vi "Sequence.CreateStepLoop.vi"(7 "Iteration":string, 8 "error in (no error)":errorcluster, 10 "Duration":dbl, 11 "Elements":T1[](array[typedef])) -> (0 "error out":errorcluster, 3 "Tasks":refnum<k24>[](array[refnum]))   [LabVIEW 2013, in "Simple Sequence Tools - Editor.lvlib"]
uses:
  Simple Sequence Tools - Editor.lvlib
  NationalInstruments.VeriStand.RealTimeSequenceDefinitionApi
  Types/Compiled.StepElementProperties.ctl
  Shared/Types/Channel.Properties.ctl
  Shared/Types/Step.Types.ctl
  Shared/SubVIs/Main.Constants.vi
  Shared/Simple Sequence Tools - Shared.lvlib
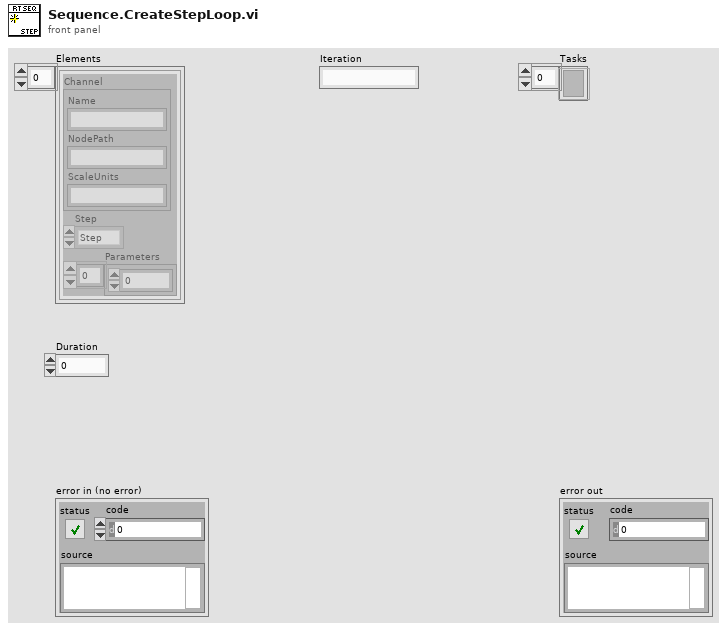
[diagram p1: front panel]
types:
  T1 = typedef "Simple Sequence Tools - Editor.lvlib/Compiled.StepElementProperties.ctl" = cluster{"Channel":T2, "Step":T3, "Parameters":dbl[]}
  T2 = typedef "Simple Sequence Tools - Shared.lvlib/Channel.Properties.ctl" = cluster{"Name":string, "NodePath":string, "ScaleUnits":string}
  T3 = typedef "Simple Sequence Tools - Shared.lvlib/Step.Types.ctl" = enum8{"Step", "iStep", "Ramp", "Unchanged", "Unknown", "Sine", "LogSine", "LinearSine", "ForcedRamp"}
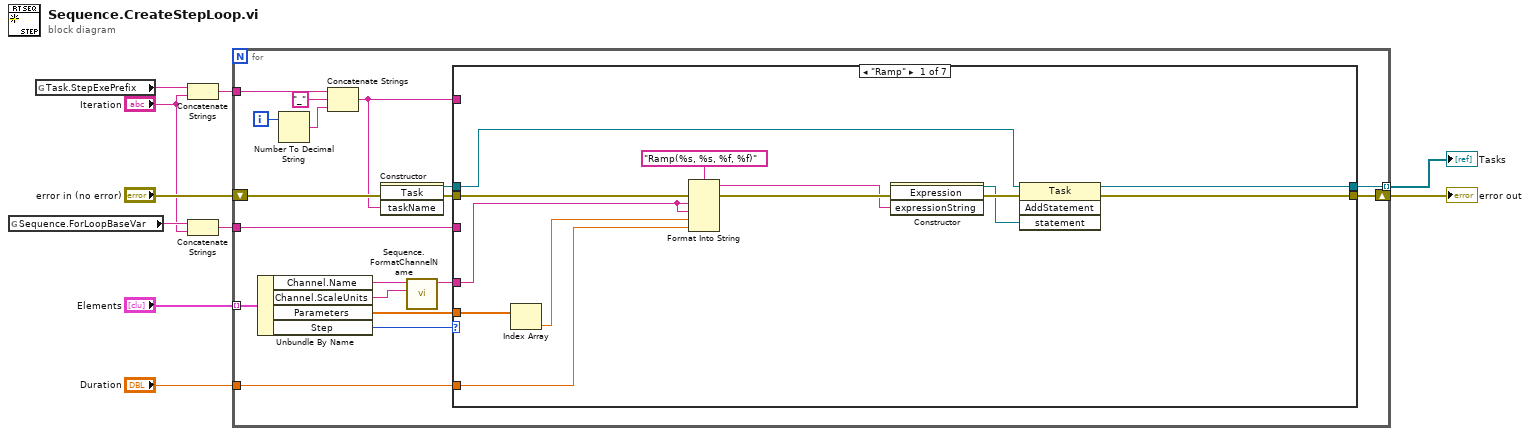
[diagram p0: block diagram]
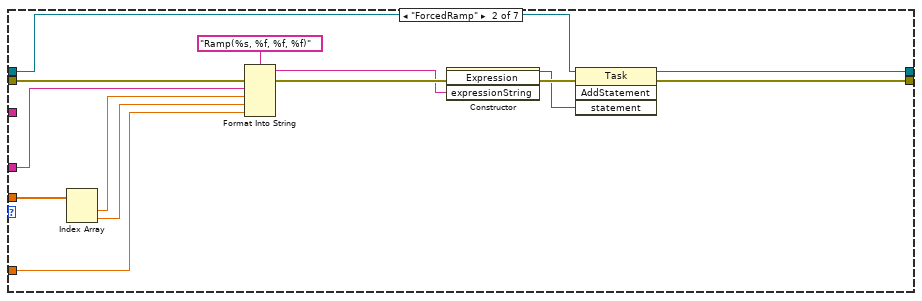
[diagram p2: hidden frame]
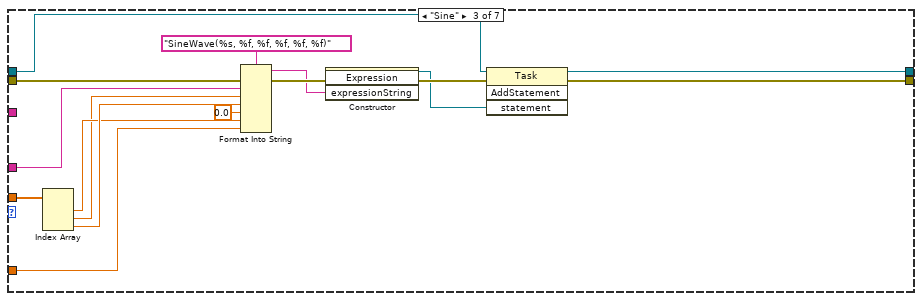
[diagram p3: hidden frame]
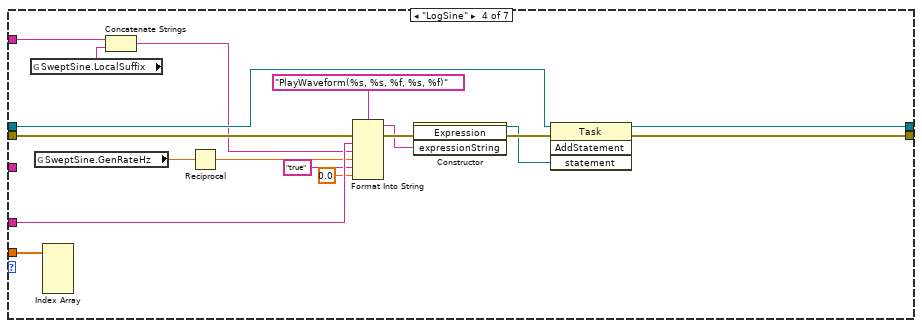
[diagram p4: hidden frame]
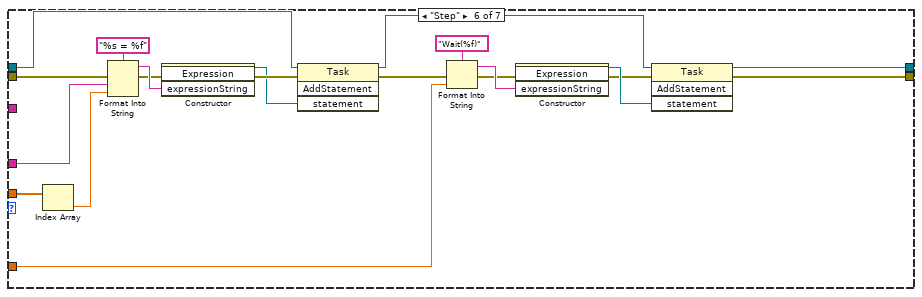
[diagram p6: hidden frame]
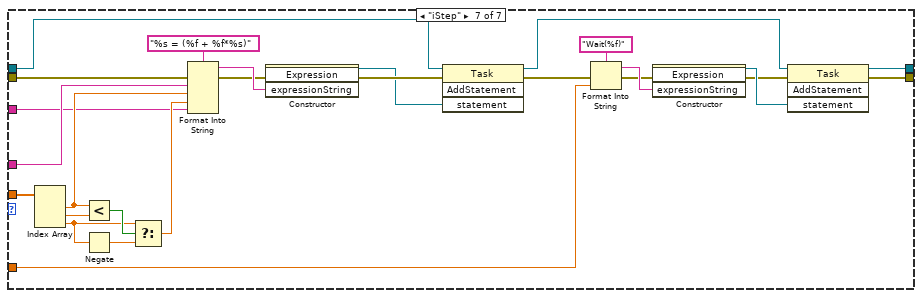
[diagram p7: hidden frame]
diagram:
  n1 = global read "Main.Constants.vi" "Sequence.ForLoopBaseVar"() -> (w3:string)
  n2 = global read "Main.Constants.vi" "Task.StepExePrefix"() -> (w5:string)
  n3 = Concatenate Strings(w5, "Iteration") -> (w4:string)
  n4 = Concatenate Strings(w3, "Iteration") -> (w1:string)
  n5 = for {
    tunnel: "Elements" -> [w24] mode=indexing
    shift-right: [w15] -> w9
    shift-left: "error in (no error)" -> [w23]
    tunnel: w4 -> [w27]
    tunnel: [w13] -> w10 mode=indexing
    tunnel: "Duration" -> [w19]
    tunnel: w1 -> [w12]
    i -> [w28]
    n6 = Unbundle By Name(w24) -> ("Channel.Name"=w22:string, "Channel.ScaleUnits"=w21:string, "Parameters"=w18:dbl[], "Step"=w17:T3)
    n7 = Number To Decimal String(number=w28) -> (decimal integer string=w25:string)  [unwired: 1 in]
    n8 = Concatenate Strings(w27, "_" ("string"), w25) -> (w11:string)
    n9 = constructor class="Task"(error in=w23, "taskName"=w11) -> (reference out=w14:refnum<k24>, error out=w16:errorcluster)  [unwired: 2 in, 2 out]
    n10 = call "Sequence.FormatChannelName.vi"("ScaleUnits"=w21, "Name"=w22) -> ("ChannelName"=w20:string)  [unwired: 9 in]
    n11 = case shown="\"Ramp\"" w17 {
      tunnel: w20 -> [w41 w55 w70 w88 _ w110 w136]
      tunnel: w18 -> [w30 w43 w69 w87 _ w109 w135]
      tunnel: w19 -> [w39 w52 w58 _ _ w100 w127]
      tunnel: [w33 w46 w63 w81 w90 w94 w121] -> w15
      tunnel: w16 -> [w38 w51 w68 w86 w90 w107 w134]
      tunnel: w14 -> [w35 w48 w65 w83 w91 w99 w126]
      tunnel: [w32 w45 w62 w80 w91 w92 w119] -> w13
      tunnel: w12 -> [_ _ _ _ _ _ w112]
      tunnel: w11 -> [_ _ _ w75 _ _ _]
      frame "Ramp" {
        n12 = Index Array(array=w30) -> (element=w40:dbl)  [unwired: 1 in]
        n13 = Format Into String(format string="Ramp(%s, %s, %f, %f)" ("expressionString"), error in=w38, w41, w41, w40, w39) -> (resulting string=w31:string, error out=w34:errorcluster)  [unwired: 1 in]
        n14 = constructor class="Expression"(error in=w34, "expressionString"=w31) -> (reference out=w36:refnum<k24>, error out=w37:errorcluster)  [unwired: 2 in, 2 out]
        n15 = invoke class="Task" method="AddStatement"(reference=w35, error in=w37, "statement"=w36) -> (reference out=w32:refnum<k24>, error out=w33:errorcluster)  [unwired: 1 in, 2 out]
      }
      frame "ForcedRamp" {
        n16 = Index Array(array=w43) -> (element #1=w54:dbl, element #2=w53:dbl)  [unwired: 2 in]
        n17 = Format Into String(format string="Ramp(%s, %f, %f, %f)" ("expressionString"), error in=w51, w55, w54, w53, w52) -> (resulting string=w44:string, error out=w47:errorcluster)  [unwired: 1 in]
        n18 = constructor class="Expression"(error in=w47, "expressionString"=w44) -> (reference out=w49:refnum<k24>, error out=w50:errorcluster)  [unwired: 2 in, 2 out]
        n19 = invoke class="Task" method="AddStatement"(reference=w48, error in=w50, "statement"=w49) -> (reference out=w45:refnum<k24>, error out=w46:errorcluster)  [unwired: 1 in, 2 out]
      }
      frame "Sine" {
        n20 = Index Array(array=w69) -> (element #1=w57:dbl, element #2=w56:dbl, element #3=w60:dbl)  [unwired: 3 in]
        n21 = Format Into String(format string="SineWave(%s, %f, %f, %f, %f, %f)" ("expressionString"), error in=w68, w70, w56, w60, 0.0 ("input 4"), w57, w58) -> (resulting string=w61:string, error out=w64:errorcluster)  [unwired: 1 in]
        n22 = constructor class="Expression"(error in=w64, "expressionString"=w61) -> (reference out=w66:refnum<k24>, error out=w67:errorcluster)  [unwired: 2 in, 2 out]
        n23 = invoke class="Task" method="AddStatement"(reference=w65, error in=w67, "statement"=w66) -> (reference out=w62:refnum<k24>, error out=w63:errorcluster)  [unwired: 1 in, 2 out]
      }
      frame "LogSine" {
        n24 = global read "Main.Constants.vi" "SweptSine.LocalSuffix"() -> (w73:string)
        n25 = global read "Main.Constants.vi" "SweptSine.GenRateHz"() -> (w72:dbl)
        n26 = Index Array(array=w87) -> ()  [unwired: 4 in, 4 out]
        n27 = Concatenate Strings(w75, w73) -> (w74:string)
        n28 = Reciprocal(x=w72) -> (1/x=w76:dbl)
        n29 = Format Into String(format string="PlayWaveform(%s, %s, %f, %s, %f)" ("expressionString"), error in=w86, w88, w74, w76, "true" ("input 4"), 0.0 ("input 4")) -> (resulting string=w79:string, error out=w82:errorcluster)  [unwired: 1 in]
        n30 = constructor class="Expression"(error in=w82, "expressionString"=w79) -> (reference out=w84:refnum<k24>, error out=w85:errorcluster)  [unwired: 2 in, 2 out]
        n31 = invoke class="Task" method="AddStatement"(reference=w83, error in=w85, "statement"=w84) -> (reference out=w80:refnum<k24>, error out=w81:errorcluster)  [unwired: 1 in, 2 out]
      }
      frame "Unchanged", Default {
      }
      frame "Step" {
        n32 = Index Array(array=w109) -> (element=w108:dbl)  [unwired: 1 in]
        n33 = Format Into String(format string="%s = %f" ("expressionString"), error in=w107, w110, w108) -> (resulting string=w104:string, error out=w95:errorcluster)  [unwired: 1 in]
        n34 = constructor class="Expression"(error in=w95, "expressionString"=w104) -> (reference out=w105:refnum<k24>, error out=w106:errorcluster)  [unwired: 2 in, 2 out]
        n35 = invoke class="Task" method="AddStatement"(reference=w99, error in=w106, "statement"=w105) -> (reference out=w93:refnum<k24>, error out=w96:errorcluster)  [unwired: 1 in, 2 out]
        n36 = Format Into String(format string="Wait(%f)", error in=w96, w100) -> (resulting string=w98:string, error out=w97:errorcluster)  [unwired: 1 in]
        n37 = constructor class="Expression"(error in=w97, "expressionString"=w98) -> (reference out=w103:refnum<k24>, error out=w102:errorcluster)  [unwired: 2 in, 2 out]
        n38 = invoke class="Task" method="AddStatement"(reference=w93, error in=w102, "statement"=w103) -> (reference out=w92:refnum<k24>, error out=w94:errorcluster)  [unwired: 1 in, 2 out]
      }
      frame "iStep" {
        n39 = Index Array(array=w135) -> (element #1=w118:dbl, element #2=w117:dbl, element #3=w114:dbl)  [unwired: 3 in]
        n40 = Less?(x=w118, y=w117) -> (x < y?=w116:bool)
        n41 = Negate(x=w114) -> (-x=w115:dbl)
        n42 = Select(t=w114, s=w116, f=w115) -> (s? t:f=w113:dbl)
        n43 = Format Into String(format string="%s = (%f + %f*%s)" ("expressionString"), error in=w134, w136, w118, w113, w112) -> (resulting string=w131:string, error out=w122:errorcluster)  [unwired: 1 in]
        n44 = constructor class="Expression"(error in=w122, "expressionString"=w131) -> (reference out=w132:refnum<k24>, error out=w133:errorcluster)  [unwired: 2 in, 2 out]
        n45 = invoke class="Task" method="AddStatement"(reference=w126, error in=w133, "statement"=w132) -> (reference out=w120:refnum<k24>, error out=w123:errorcluster)  [unwired: 1 in, 2 out]
        n46 = Format Into String(format string="Wait(%f)", error in=w123, w127) -> (resulting string=w125:string, error out=w124:errorcluster)  [unwired: 1 in]
        n47 = constructor class="Expression"(error in=w124, "expressionString"=w125) -> (reference out=w130:refnum<k24>, error out=w129:errorcluster)  [unwired: 2 in, 2 out]
        n48 = invoke class="Task" method="AddStatement"(reference=w120, error in=w129, "statement"=w130) -> (reference out=w119:refnum<k24>, error out=w121:errorcluster)  [unwired: 1 in, 2 out]
      }
    }
  }
  "Tasks" <- w10
  "error out" <- w9
